vi "Main.vi"() -> ()   [LabVIEW 2021]
uses:
  Classes/Communication/Comm/Comm.lvclass
  Classes/Communication/Serial/Serial.lvclass
  Classes/Communication/Wifi/Wifi.lvclass
panel:
  in  "Stop":bool
  out "Sensor Reading":dbl(graph)
  in  "Write":string
  out "Read":string
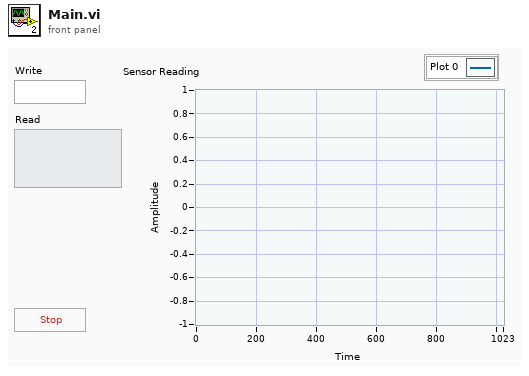
[diagram p1: front panel]
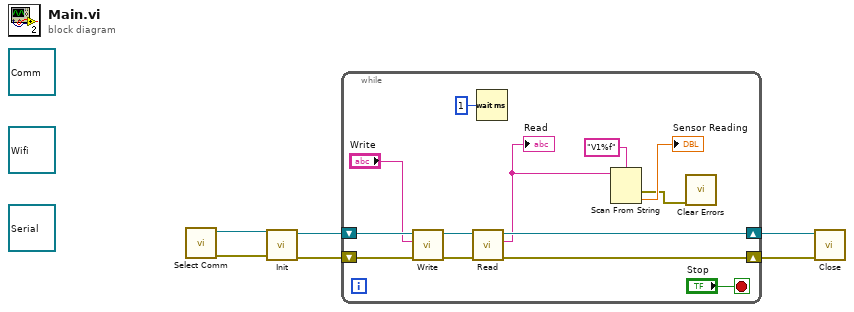
[diagram p0: block diagram]
diagram:
  (unwired) refnum<class "Wifi.lvclass"> refnum ("Wifi.lvclass")
  (unwired) refnum<class "Serial.lvclass"> refnum ("Serial.lvclass")
  (unwired) refnum<class "Comm.lvclass"> refnum ("Comm in")
  n1 = call "Select Comm.vi"() -> ("error out"=w1:errorcluster, "Comm.lvclass"=w2:refnum<class "Comm.lvclass">)  [unwired: 10 in]
  n2 = call-dynamic "Init.vi"("error in (no error)"=w1, "Comm in"=w2) -> ("error out"=w6:errorcluster, "Comm out"=w3:refnum<class "Comm.lvclass">)  [unwired: 8 in]
  n3 = while {
    shift-right: [w17] -> w4
    shift-left: w6 -> [w19]
    shift-right: [w18] -> w5
    shift-left: w3 -> [w15]
    stop <- "Stop" stop-if-true
    n4 = call-dynamic "Write.vi"("error in (no error)"=w19, "Message"="Write", "Comm in"=w15) -> ("error out"=w16:errorcluster, "Comm out"=w14:refnum<class "Comm.lvclass">)  [unwired: 7 in]
    n5 = call-dynamic "Read.vi"("error in (no error)"=w16, "Comm in"=w14) -> ("error out"=w17:errorcluster, "Message"=w11:string, "Comm out"=w18:refnum<class "Comm.lvclass">)  [unwired: 7 in]
    "Read" <- w11
    n6 = Wait (ms)(milliseconds to wait=u32 1) -> ()  [unwired: 1 out]
    n7 = Scan From String(format string="V1%f", input string=w11) -> (error out=w7:errorcluster, output 1=→"Sensor Reading":dbl)  [unwired: 3 in, 2 out]
    n8 = call <vilib>:"Clear Errors.vi"("error in (no error)"=w7) -> ()  [unwired: 5 in, 2 out]
  }
  n9 = call-dynamic "Close.vi"("error in (no error)"=w4, "Comm in"=w5) -> ()  [unwired: 8 in, 2 out]
